vi "Dispose Shared Variables Host.vi"(8 "error in (no error)":errorcluster, 11 "Shared Variable References":T1) -> (0 "error out":errorcluster)   [LabVIEW 2015]
doc: "This VI closes the references to the application shared variables."
uses:
  Custom Controls/Display State.ctl
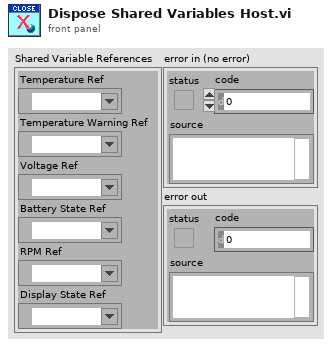
[diagram p1: front panel]
types:
  T1 = cluster{"Temperature Ref":refnum<k21>, "Temperature Warning Ref":refnum<k21>, "Voltage Ref":refnum<k21>, "Battery State Ref":refnum<k21>, "RPM Ref":refnum<k21>, "Display State Ref":refnum<k21>}
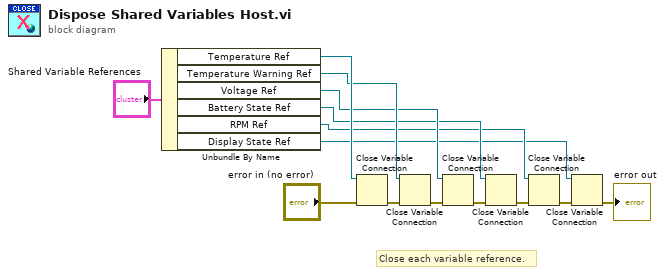
[diagram p0: block diagram]
diagram:
  # "Close each variable reference."
  n1 = Unbundle By Name("Shared Variable References") -> ("Temperature Ref"=w13:refnum<k21>, "Temperature Warning Ref"=w12:refnum<k21>, "Voltage Ref"=w11:refnum<k21>, "Battery State Ref"=w10:refnum<k21>, "RPM Ref"=w9:refnum<k21>, "Display State Ref"=w8:refnum<k21>)
  n2 = Close Variable Connection(8:"error in (no error)", 11:w13) -> (0:w6:errorcluster)
  n3 = Close Variable Connection(8:w6, 11:w12) -> (0:w5:errorcluster)
  n4 = Close Variable Connection(8:w5, 11:w11) -> (0:w4:errorcluster)
  n5 = Close Variable Connection(8:w4, 11:w10) -> (0:w3:errorcluster)
  n6 = Close Variable Connection(8:w3, 11:w9) -> (0:w2:errorcluster)
  n7 = Close Variable Connection(8:w2, 11:w8) -> (0:→"error out":errorcluster)
